vi "Insert.vi"(8 "error in (no error)":errorcluster, 9 "Item":refnum<class>, 10 "Index":i32, 11 "BufferedArray in":refnum<class "BufferedArray.lvclass">) -> (0 "error out":errorcluster, 3 "BufferedArray out":refnum<class "BufferedArray.lvclass">)   [LabVIEW 2017, in "LapDog.Collections.v0.Lists.Implementations.lvlib" / "BufferedArray.lvclass"]
uses:
  BufferedArray.lvclass
  BufferedArray.lvclass/BufferedArray.ctl
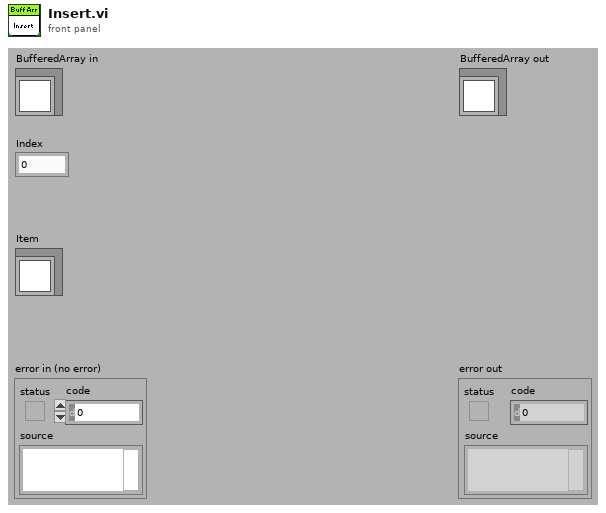
[diagram p1: front panel]
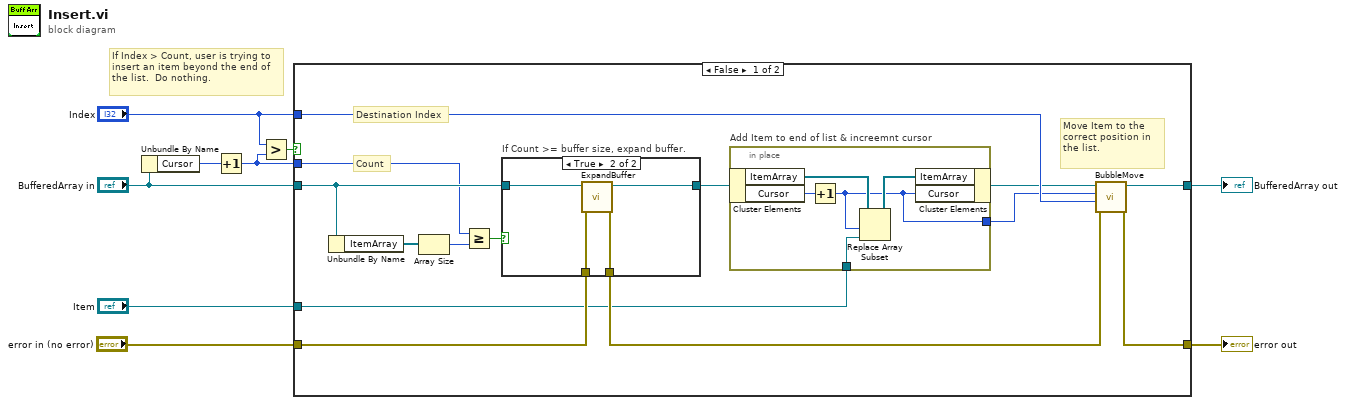
[diagram p0: block diagram]
diagram:
  # "If Index > Count, user is trying to insert an item beyond the end of the list.  Do nothing."
  n1 = Unbundle By Name("BufferedArray in") -> ("Cursor"=w2:i32)
  n2 = Increment(x=w2) -> (x+1=w4:i32)
  n3 = Greater?(x="Index", y=w4) -> (0:w5:bool)
  n4 = case shown="False" w5 {
    tunnel: [w17 w36] -> w9
    tunnel: "error in (no error)" -> [w20 w35]
    tunnel: [w15 w35] -> w7
    tunnel: "BufferedArray in" -> [w19 w36]
    tunnel: w4 -> [w18 _]
    tunnel: "Index" -> [w14 _]
    tunnel: "Item" -> [w11 _]
    frame False {
      # "Move Item to the correct position in the list."
      # "Destination Index"
      # "Count"
      n5 = Unbundle By Name(w19) -> ("ItemArray"=w23:refnum<class>[])
      n6 = Array Size(array=w23) -> (size(s)=w22:i32)
      n7 = Greater Or Equal?(x=w18, y=w22) -> (x >= y?=w21:bool)
      n8 = case "If Count >= buffer size, expand buffer." shown="True" w21 {
        tunnel: w19 -> [w30 w34]
        tunnel: [w30 w33] -> w13
        tunnel: w20 -> [w29 w32]
        tunnel: [w29 w31] -> w16
        frame False {
        }
        frame True {
          n9 = call-dynamic "ExpandBuffer.vi"("error in (no error)"=w32, "BufferedArray in"=w34) -> ("error out"=w31:errorcluster, "BufferedArray out"=w33:refnum<class "BufferedArray.lvclass">)  [unwired: 8 in]
        }
      }
      n10 = in-place "Add Item to end of list & increemnt cursor" {
        in-place-border: w11 -> [w25]
        in-place-border: [w24] -> w10
        n11 = in-place-cluster #1(w13) -> ("ItemArray"=w28:refnum<class>[], "Cursor"=w26:i32)
        n12 = Increment(x=w26) -> (x+1=w24:i32)
        n13 = Replace Array Subset(array=w28, new element=w25, index=w24) -> (w27:refnum<class>[])
        n14 = in-place-cluster #1("ItemArray"=w27, "Cursor"=w24) -> (w12:refnum<class "BufferedArray.lvclass">)
      }
      n15 = call "BubbleMove.vi"("error in (no error)"=w16, "Destination Index"=w14, "Current Index"=w10, "BufferedArray in"=w12) -> ("error out"=w15:errorcluster, "BufferedArray out"=w17:refnum<class "BufferedArray.lvclass">)  [unwired: 6 in]
    }
    frame True {
    }
  }
  "error out" <- w7
  "BufferedArray out" <- w9
